vi "CANopen read.vi"() -> ()   [LabVIEW 2017]
uses:
  <vilib>/CANopenLib/CANOPEN.llb/CANopen BaudRate.ctl
  <vilib>/CANopenLib/CANOPEN.llb/CANopen Interface Create.vi
  <vilib>/CANopenLib/CANOPEN.llb/CANopen SDO Create.vi
  <vilib>/CANopenLib/CANOPEN.llb/CANopen SDO Read [U32].vi
panel:
  in  "node-ID":u8
  in  "object sub-index (0)":u8 format="%.0x"
  in  "object index":u16 format="%.0x"
  out "U32 data":u32
  out "description":string
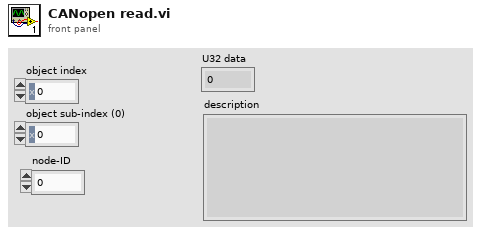
[diagram p1: front panel]
types:
  T1 = typedef "CANopen BaudRate.ctl" = u32
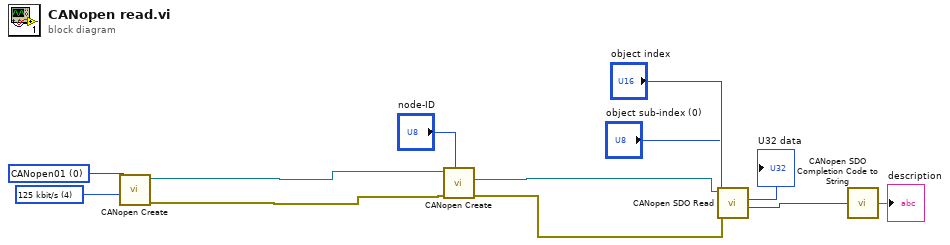
[diagram p0: block diagram]
diagram:
  w11 = T1 4 items=["1 Mbit/s"=0, "800 kbit/s"=1, "500 kbit/s"=2, "250 kbit/s"=3, "125 kbit/s"=4, "50 kbit/s"=6, "20 kbit/s"=7, "10 kbit/s"=8] ("baud rate")
  w12 = u32 0 items=["CANopen01", "CANopen02", "CANopen03", "CANopen04", "CANopen05", "CANopen06", "CANopen07", "CANopen08", "CANopen09", "CANopen10", "CANopen11", "CANopen12", "CANopen13", "CANopen14", "CANopen15", "CANopen16", "CANopen17", "CANopen18", "CANopen19", "CANopen20", "CANopen21", "CANopen22", "CANopen23", "CANopen24", "CANopen25", "CANopen26", "CANopen27", "CANopen28", "CANopen29", "CANopen30", "CANopen31", "CANopen32"] ("interface name")
  n1 = call-poly <vilib>:"CANopen Create.vi"("baud rate"=w11, "interface name"=w12) -> ("error out"=w8:errorcluster, "interface object out"=w7:refnum<k20>)  [unwired: 8 in]
  n2 = call-poly <vilib>:"CANopen Create.vi"("node-ID"="node-ID", "error in (no error)"=w8, "interface object in"=w7) -> ("error out"=w10:errorcluster, "SDO object out"=w9:refnum<k20>)  [unwired: 6 in, 1 out]
  n3 = call-poly <vilib>:"CANopen SDO Read.vi"("error in (no error)"=w10, "object sub-index (0)"="object sub-index (0)", "object index"="object index", "SDO object in"=w9) -> ("completion code"=w6:u32, "U32 data"=→"U32 data":u32)  [unwired: 4 in, 2 out]
  n4 = call <vilib>:"CANopen SDO Completion Code to String.vi"("SDO completion code"=w6) -> ("description"=→"description":string)
